vi "Read Change Instrument Event.vi"(8 "error in (no error)":errorcluster, 11 "Engine in":refnum<class "Engine.lvclass">) -> (0 "error out":errorcluster, 2 "Change Instrument Event":refnum<user-event>, 3 "Engine out":refnum<class "Engine.lvclass">)   [LabVIEW 2019, in "Engine.lvlib" / "Engine.lvclass"]
uses:
  Project/Engine.lvclass
  Project/Engine.lvclass/Engine.ctl
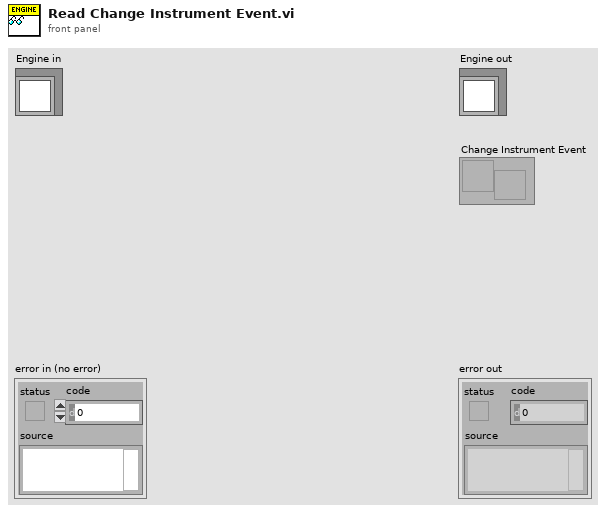
[diagram p1: front panel]
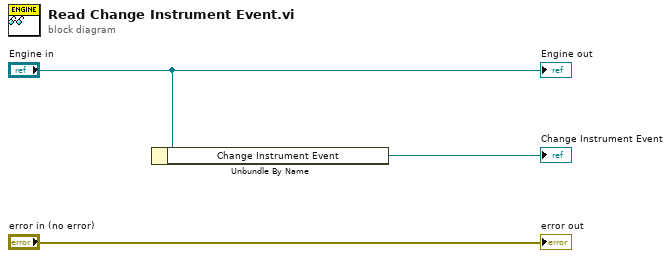
[diagram p0: block diagram]
diagram:
  n1 = Unbundle By Name("Engine in") -> ("Change Instrument Event"=→"Change Instrument Event":refnum<user-event>)
  "error out" <- "error in (no error)"
  "Engine out" <- "Engine in"
